vi "Control Panel TeleOp.vi"(7 "Gamepad":T1={"A"=FALSE, "B"=FALSE, "X"=FALSE, "Y"=FALSE, "LB"=FALSE, "RB"=FALSE, "Back"=FALSE, "Next"=FALSE, "Left Stick X"=0.0, "Left Stick Y"=0.0, "Right Stick X"=0.0, "Right Stick Y"=0.0, "LT"=1.0, "RT"=1.0, "D-Pad X"=0, "D-Pad Y"=0} {"Left Stick X" scale=-1.0..1.0; "Left Stick Y" scale=1.0..-1.0; "Right Stick X" scale=-1.0..1.0; "Right Stick Y" scale=1.0..-1.0; "D-Pad Y" step=1 scale=1.0..-1.0; "D-Pad X" step=1 scale=-1.0..1.0; "LT" scale=1.0..-1.0; "RT" scale=1.0..-1.0}, 9 "Color":T2, 10 "Arm Out":bool, 11 "Arm In":bool) -> (0 "Game Data":string, 2 "Wheel":dbl(slide) scale=-1.0..1.0, 3 "Arm":dbl(slide) scale=-1.0..1.0)   [LabVIEW 2019]
uses:
  Support/Color.ctl
  Support/Gamepad.ctl
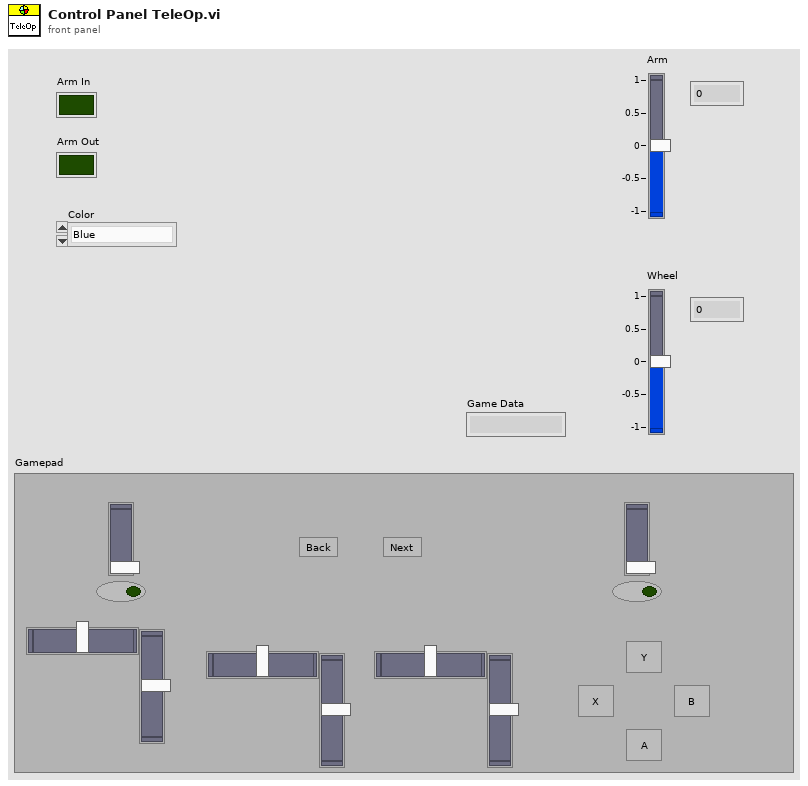
[diagram p1: front panel]
types:
  T1 = typedef "Gamepad.ctl" = cluster{"A":bool, "B":bool, "X":bool, "Y":bool, "LB":bool, "RB":bool, "Back":bool, "Next":bool, "Left Stick X":dbl, "Left Stick Y":dbl, "Right Stick X":dbl, "Right Stick Y":dbl, "LT":dbl, "RT":dbl, "D-Pad X":i32, "D-Pad Y":i32}
  T2 = typedef "Color.ctl" = enum16{"Blue", "Green", "Red", "Yellow"}
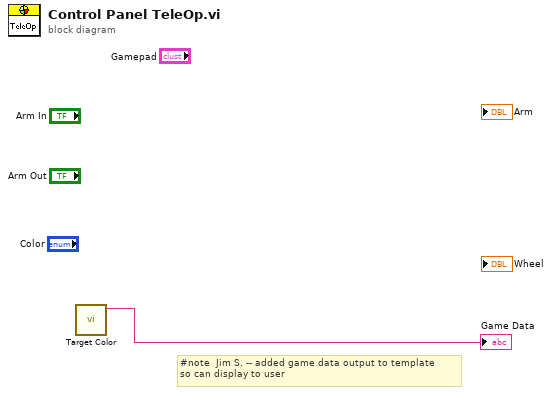
[diagram p0: block diagram]
diagram:
  # "#note  Jim S. -- added game data output to template\nso can display to user"
  n1 = call "Target Color.vi"() -> ("Color"=→"Game Data":string)  [unwired: 11 in]
